vi "Status.vi"(8 "Error In":errorcluster) -> (0 "Error Out":errorcluster)   [LabVIEW 2017, in "Tests.lvlib" / "Reader.lvlib"]
uses:
  Reader.lvlib
  src/LabPack/Public/Controls/Status.ctl
  src/LabPack/Public/Reader/Reader.lvclass/Reader.ctl
  <vilib>/addons/_JKI Toolkits/Caraya/classes/Test/Test.lvclass
  src/LabPack/Public/Reader/Reader.lvclass
  <vilib>/addons/_JKI Toolkits/Caraya/classes/Assert/Assert.lvclass
  src/LabPack/LabPack.lvlib
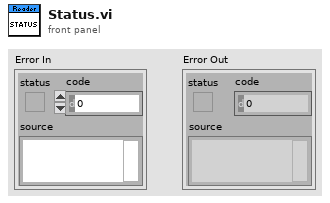
[diagram p1: front panel]
types:
  T1 = typedef "LabPack.lvlib/Status.ctl" = enum32{"OK", "Out of Memory", "Null Value", "Encoder"}
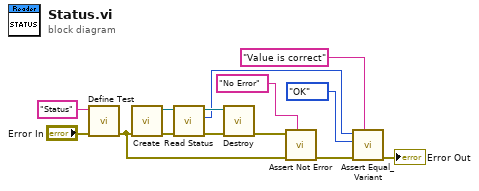
[diagram p0: block diagram]
diagram:
  n1 = call <vilib>:"Define Test.vi"("error in (no error)"="Error In", "Label (VI Title)"="Status") -> ("error out"=w4:errorcluster)  [unwired: 9 in]
  n2 = call "Create.vi"("Error In"=w4) -> ("Error Out"=w11:errorcluster, "Reader"=w12:refnum<class "Reader.lvclass">)  [unwired: 9 in]
  n3 = call "Read Status.vi"("Error In"=w11, "Reader In"=w12) -> ("Error Out"=w9:errorcluster, "Status"=w2:T1, "Reader Out"=w10:refnum<class "Reader.lvclass">)  [unwired: 7 in]
  n4 = call "Destroy.vi"("Error In"=w9, "Reader"=w10) -> ("Error Out"=w8:errorcluster)  [unwired: 9 in]
  n5 = call <vilib>:"Assert Not Error.vi"("Label"="No Error", "error in (no error)"=w4, "Not Error?"=w8) -> ("error out"=w5:errorcluster)  [unwired: 8 in]
  n6 = call <vilib>:"Assert Equal_Variant.vi"("Label"="Value is correct", "error in (no error)"=w5, "Y"=Status."OK" ("Status"), "X"=w2) -> ("error out"=→"Error Out":errorcluster)  [unwired: 7 in]
